vi "Onboard AIs Global.vi"() -> ()   [LabVIEW 2013]
panel:
  out "Onboard AI's":fxp<+/-,28,17>[](array[numeric])
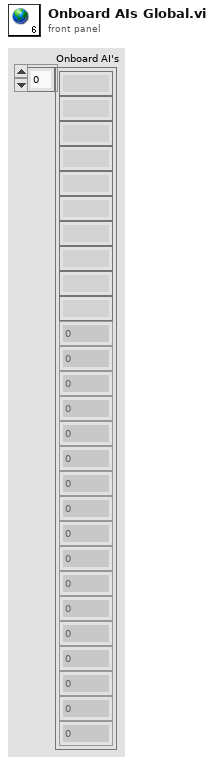
[diagram p1: front panel]
diagram:
